vi "DigitalInOut_write.vi"(8 "error in (no error)":errorcluster, 10 "value":bool, 11 "DigitalInOut in":refnum<class "DigitalInOut.lvclass">) -> (0 "error out":errorcluster, 3 "DigitalInOut out":refnum<class "DigitalInOut.lvclass">)   [LabVIEW 2011, in "mbed_LVLibrary.lvlib" / "DigitalInOut.lvclass"]
uses:
  DigitalInOut.lvclass
  DigitalInOut.lvclass/DigitalInOut.ctl
  Transport Mechanisms/mbed/mbed.lvclass
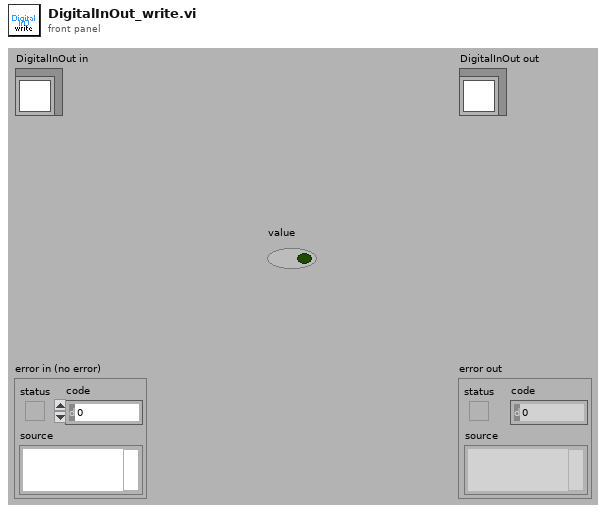
[diagram p1: front panel]
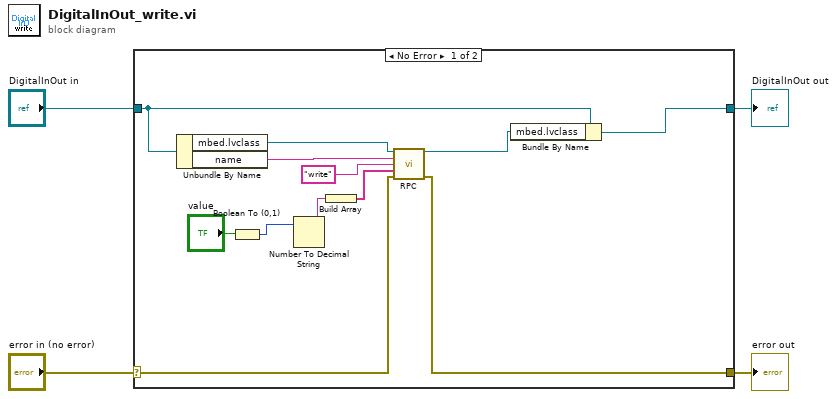
[diagram p0: block diagram]
diagram:
  n1 = case shown="No Error" "error in (no error)" {
    selector: "error in (no error)" -> [w6 w18]
    tunnel: [w5 w18] -> w3
    tunnel: [w8 w17] -> w1
    tunnel: "DigitalInOut in" -> [w9 w17]
    frame No Error {
      n2 = Unbundle By Name(w9) -> ("mbed.lvclass"=w16:refnum<class "mbed.lvclass">, "name"=w15:string)
      n3 = Boolean To (0,1)(Boolean="value") -> (0, 1=w11:i16)
      n4 = Number To Decimal String(number=w11) -> (decimal integer string=w10:string)  [unwired: 1 in]
      n5 = Build Array(w10) -> (w13:string[])
      n6 = call-dynamic "RPC.vi"("mbed in"=w16, "Name"=w15, "method"="write", "Args"=w13, "error in (no error)"=w6) -> ("mbed out"=w7:refnum<class "mbed.lvclass">, "error out"=w5:errorcluster)  [unwired: 8 in, 1 out]
      n7 = Bundle By Name(cluster=w9, "mbed.lvclass"=w7) -> (w8:refnum<class "DigitalInOut.lvclass">)
    }
    frame Error {
    }
  }
  "error out" <- w3
  "DigitalInOut out" <- w1
